vi "ADC_kernal_server.vi"(0 "Board type":T2=enum."Local ADAM", 1 "interval scanning":bool, 2 "Client Time":dbl, 5 "No of samples+extra":i32=128 min=0 step=1, 7 "Trigger mode":T1, 9 "output polarity":u16(ring)=1 items=["do not change", "positive", "negative"], 11 "Ch & spans":T3[](array[typedef]) {"low limit (-10V)" format="%.3f"; "high limit (10V)" format="%.3f"}, 12 "Actual Sampling rate (Hz)":dbl=1000.0 format="%.2f", 13 "Local Client?":bool, 14 "Current Block No":i32) -> (4 "I16 data":i16[][](array[numeric]), 6 "Block Timings":T4={"Started"=0.0, "Ended"=0.0, "Analogue Frequency Hz"=1000.0} {"Analogue Frequency Hz" format="%.2f"}, 10 "group channel settings":T5(array[cluster]) {"scale offset" format="%.2f"; "scale multiplier" format="%.2f"; "gain" format="%.2f"; "range" format="%.2f"; "lower input limits" format="%.2f"; "upper input limits" format="%.2f"}, 15 "error out":errorcluster)   [LabVIEW 2010]
uses:
  Controls/Block_start_and_end.ctl
  Controls/Ch_and_Spans.ctl
  Controls/Board_Types.ctl
  Controls/Trigger_Mode.ctl
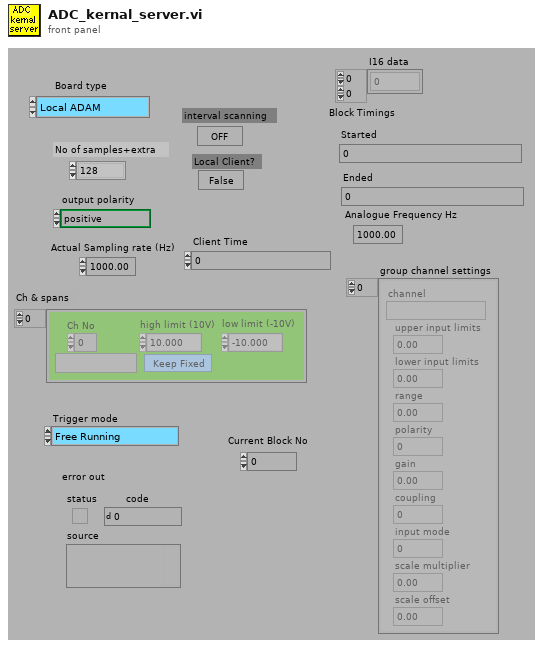
[diagram p1: front panel]
types:
  T1 = typedef "Trigger_Mode.ctl" = enum16{"Free Running", "Start on Trigger", "Trigger Every Block", "Trigger Every Sample"}
  T2 = typedef "Board_Types.ctl" = enum16{"Simulate", "Local ADAM", "Server ADAM", "NI-DAQmx", "NI-DAQmxBase", "ADC488", "DT LV-link"}
  T3 = typedef "Ch_and_Spans.ctl" = cluster{"high limit (10V)":sgl, "low limit (-10V)":sgl, "Ch No":i16, "Var name":string, "Use Latest Calib":bool}
  T4 = typedef "Block_start_and_end.ctl" = cluster{"Started":dbl, "Ended":dbl, "Analogue Frequency Hz":dbl}
  T5 = cluster{"channel":string, "upper input limits":sgl, "lower input limits":sgl, "range":sgl, "polarity":u16, "gain":sgl, "coupling":u16, "input mode":u16, "scale multiplier":dbl, "scale offset":dbl}[]
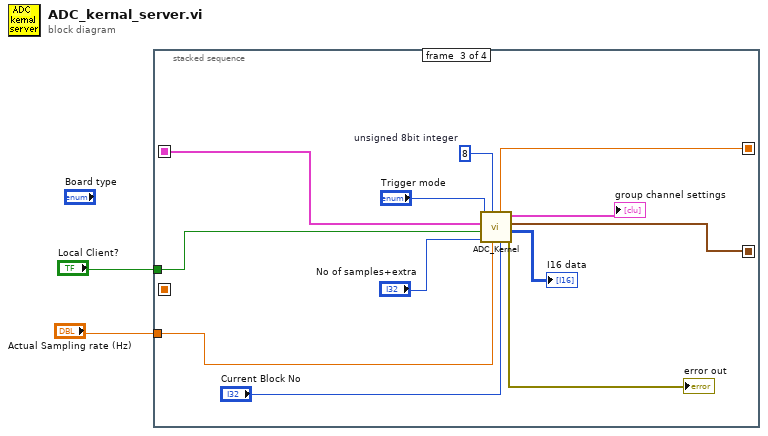
[diagram p0: block diagram]
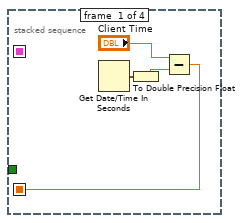
[diagram p2: hidden frame]
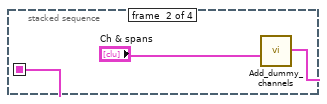
[diagram p3: hidden frame]
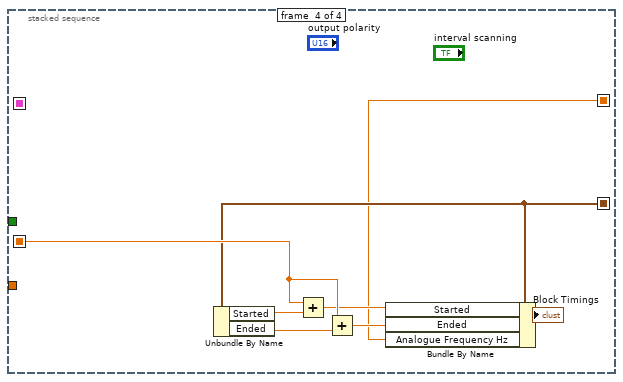
[diagram p4: hidden frame]
diagram:
  n1 = stacked-sequence {
    seq-local: [_ w8 _ _] -> [_ _ w15 _]
    seq-local: [w4 _ _ _] -> [_ _ _ w27]
    seq-local: [_ _ w17 _] -> [_ _ _ w22]
    seq-local: [_ _ w9 _] -> [_ _ _ w21]
    tunnel: "Actual Sampling rate (Hz)" -> [_ _ w13 _]
    tunnel: "Local Client?" -> [_ _ w14 _]
    frame #0 {
      n2 = Get Date/Time In Seconds() -> (seconds since 1Jan1904=w3:timestamp)
      n3 = To Double Precision Float(number=w3) -> (double precision float=w5:dbl)
      n4 = Subtract(x="Client Time", y=w5) -> (x-y=w4:dbl)
    }
    frame #1 {
      n5 = call "Add_dummy_channels.vi"("Ch & spans"="Ch & spans") -> ("Ch & spans"=w8:T3[])
    }
    frame #2 {
      w20 = u8 8  # unsigned 8bit integer
      n6 = call "ADC_Kernel.vi"("Current Block No"="Current Block No", "Sampling rate (Hz)"=w13, "GPIB Address"=w20, "No of samples"="No of samples+extra", "Local Client?"=w14, "Ch & spans"=w15, "Trigger mode"="Trigger mode") -> ("error out (no error)"=→"error out":errorcluster, "Binary array"=→"I16 data":i16[][], "Block Timings"=w17:T4, "group channel settings"=→"group channel settings":T5, "Actual Sampling rate (Hz)"=w9:dbl)
    }
    frame #3 {
      n7 = Unbundle By Name(w22) -> ("Started"=w26:dbl, "Ended"=w25:dbl)
      n8 = Add(x=w27, y=w26) -> (x+y=w23:dbl)
      n9 = Add(x=w27, y=w25) -> (x+y=w24:dbl)
      n10 = Bundle By Name(cluster=w22, "Started"=w23, "Ended"=w24, "Analogue Frequency Hz"=w21) -> (→"Block Timings":T4)
    }
  }
